vi "test Add Script Deploy.vi"(8 "error in":errorcluster, 11 "TestCase in":refnum<class "Examples.lvclass">) -> (0 "error out":errorcluster, 3 "TestCase out":refnum<class "Examples.lvclass">)   [LabVIEW 2020, in "Examples.lvclass"]
uses:
  Examples.lvclass
  <vilib>/addons/_JKI Toolkits/VI Tester/TestCase.llb/TestCase.lvclass
  7f6914e5-79d7-41a5-a6cd-be6651e4326d.vi
  C:/git/ni/niveristand-custom-device-testing-tools/VeriStandTestCase/VeriStandTestCase.lvclass
  C:/Program Files (x86)/National Instruments/LabVIEW 2020/vi.lib/addons/_JKI Toolkits/VI Tester/TestCase.llb/TestCase.lvclass
  C:/git/ni/niveristand-aim-arinc429-custom-device/Source/Scripting Examples/Tests/Examples.lvclass
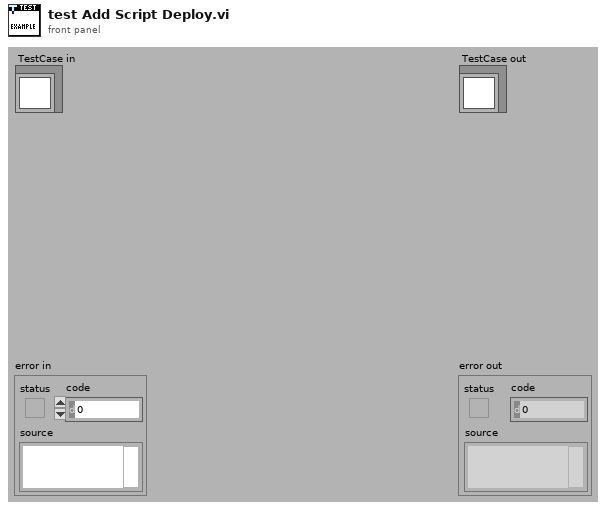
[diagram p1: front panel]
types:
  T1 = typedef "NI_VS Workspace ExecutionAPI.lvlib/WorkspaceAPI.ctl" = refnum<k24>
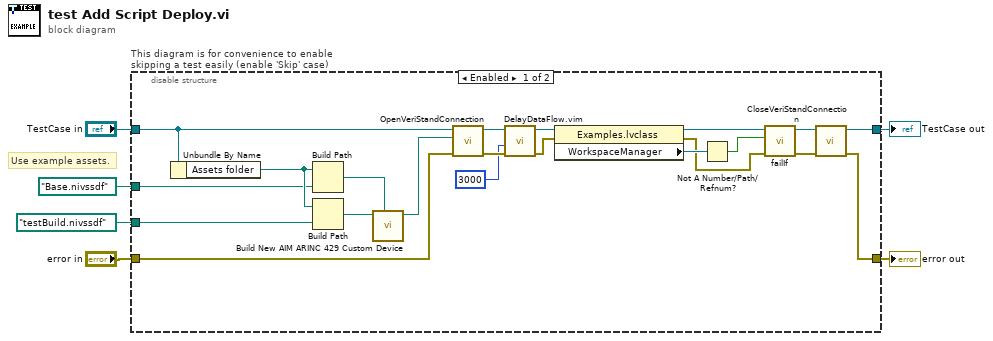
[diagram p0: block diagram]
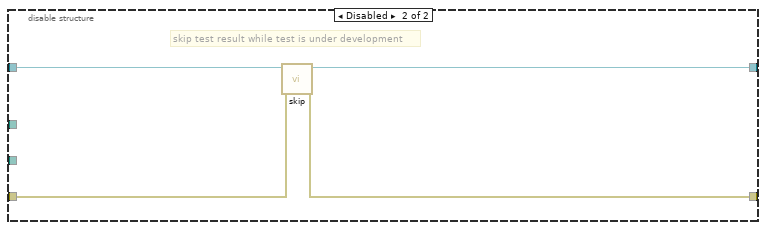
[diagram p2: hidden frame]
diagram:
  # "Use example assets."
  n1 = disable-structure "This diagram is for convenience to enable skipping a test easily (enable 'Skip' case)" shown="Enabled" {
    disable-tunnel: "TestCase in" -> [w14 w30]
    disable-tunnel: [w15 w28] -> w3
    disable-tunnel: [w16 w29] -> w5
    disable-tunnel: "error in" -> [w7 w27]
    disable-tunnel: path "testBuild.nivssdf" ("name or relative path") -> [w13 _]
    disable-tunnel: path "Base.nivssdf" ("name or relative path") -> [w10 _]
    frame Enabled {
      n2 = Unbundle By Name(w14) -> ("Assets folder"=w11:path)
      n3 = Build Path(base path=w11, name or relative path=w10) -> (appended path=w9:path)
      n4 = Build Path(base path=w11, name or relative path=w13) -> (appended path=w12:path)
      n5 = call "Build New AIM ARINC 429 Custom Device.vi"("Base System Definition File"=w9, "Output System Definition File"=w12) -> ("AIM ARINC 429 System Definition"=w8:path)  [unwired: 9 in]
      n6 = call-dynamic "OpenVeriStandConnection.vi"("error in (no error)"=w7, "System Definition File"=w8, "VeriStand Test Case in"=w14) -> ("error out"=w19:errorcluster, "VeriStand Test Case out"=w18:refnum<class "Examples.lvclass">)  [unwired: 6 in, 1 out]
      n7 = call "DelayDataFlow.vim"("value in"=w19, "milliseconds to wait"=u32 3000) -> ("value out"=w26:errorcluster)  [unwired: 2 in, 1 out]
      n8 = property class="Examples.lvclass"(reference=w18, error in=w26) -> (reference out=w25:refnum<class "Examples.lvclass">, error out=w20:errorcluster, "WorkspaceManager"=w22:T1)
      n9 = Not A Number/Path/Refnum?(number/path/refnum=w22) -> (NaN/Path/Refnum?=w21:bool)
      n10 = call-dynamic "failIf.vi"("error in (no error)"=w20, "fail"=w21, "TestCase in"=w25) -> ("error out"=w23:errorcluster, "TestCase out"=w24:refnum<class "Examples.lvclass">)  [unwired: 7 in]
      n11 = call-dynamic "CloseVeriStandConnection.vi"("error in (no error)"=w23, "VeriStand Test Case in"=w24) -> ("error out"=w16:errorcluster, "VeriStand Test Case out"=w15:refnum<class "Examples.lvclass">)  [unwired: 8 in]
    }
    frame Disabled {
      # "skip test result while test is under development"
      n12 = call <vilib>:"skip.vi"("error in (no error)"=w27, "TestCase in"=w30) -> ("error out"=w29:errorcluster, "TestCase out"=w28:refnum<class "Examples.lvclass">)  [unwired: 8 in]
    }
  }
  "error out" <- w5
  "TestCase out" <- w3
